vi "Pattern Rotation.vi"(1 "Rotation array":T1(array[cluster]), 2 "Rotation(degree)":dbl, 3 "Inkscape Image Size":cluster{"Width":dbl, "Height":dbl}) -> (0 "Rotated array":T1(array[cluster]))   [LabVIEW 2013]
uses:
  <vilib>/Analysis/coordinate.llb/2D Cartesian Coordinate Shift (Array).vi
  <vilib>/Analysis/coordinate.llb/2D Cartesian Coordinate Rotation (Array).vi
  <vilib>/Analysis/NI_AALPro.lvlib
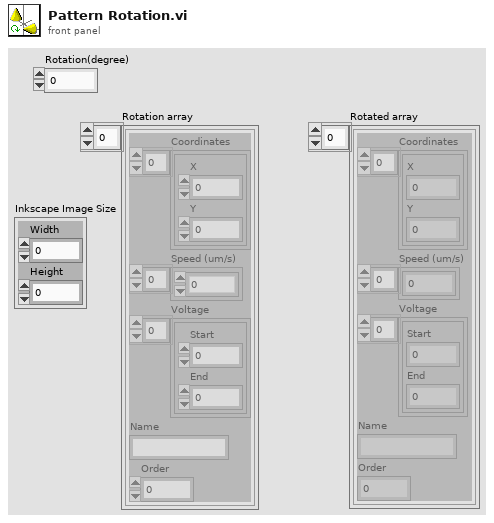
[diagram p1: front panel]
types:
  T1 = cluster{"Coordinates":cluster{"X":dbl, "Y":dbl}[], "Speed (um/s)":dbl[], "Voltage":cluster{"Start":dbl, "End":dbl}[], "Name":string, "Order":i32}[]
  T2 = cluster{"Coordinates":cluster{"X":dbl, "Y":dbl}[], "Speed (um/s)":dbl[], "Voltage":cluster{"Start":dbl, "End":dbl}[], "Name":string, "Order":i32}
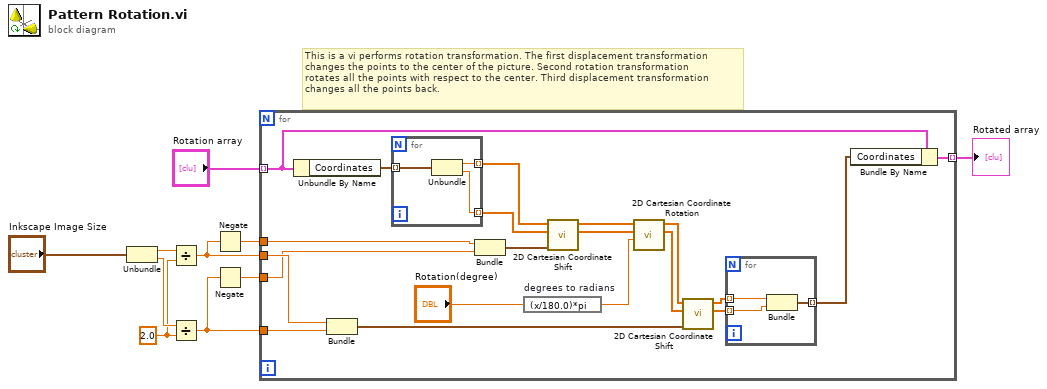
[diagram p0: block diagram]
diagram:
  w8 = 2.0 ("y")
  # "This is a vi performs rotation transformation. The first displacement transformation\nchanges the points to the center of the picture. Second rotation transformation \nrotates all the points with respect to the center. Third displacement transformation\nchanges all the points back."
  n1 = Unbundle("Inkscape Image Size") -> ("Width"=w10:dbl, "Height"=w9:dbl)
  n2 = Divide(x=w10, y=w8) -> (x/y=w6:dbl)
  n3 = Divide(x=w9, y=w8) -> (x/y=w4:dbl)
  n4 = Negate(x=w6) -> (-x=w7:dbl)
  n5 = Negate(x=w4) -> (-x=w5:dbl)
  n6 = for {
    tunnel: w7 -> [w30]
    tunnel: w6 -> [w29]
    tunnel: w5 -> [w28]
    tunnel: w4 -> [w27]
    tunnel: "Rotation array" -> [w13] mode=indexing
    tunnel: [w11] -> w1 mode=indexing
    n7 = Unbundle By Name(w13) -> ("Coordinates"=w16:cluster{"X":dbl, "Y":dbl}[])
    n8 = Bundle(w29, w27) -> (w19:cluster{dbl, dbl})  [unwired: 1 in]
    n9 = for {
      tunnel: w16 -> [w33] mode=indexing
      tunnel: [w32] -> w15 mode=indexing
      tunnel: [w31] -> w14 mode=indexing
      n10 = Unbundle(w33) -> ("X"=w32:dbl, "Y"=w31:dbl)
    }
    n11 = Bundle(w30, w28) -> (w20:cluster{dbl, dbl})  [unwired: 1 in]
    n12 = expression code="(x/180.0)*pi" "degrees to radians"("Rotation(degree)") -> (w17:dbl)
    n13 = call-poly <vilib>:"2D Cartesian Coordinate Shift.vi"("shift"=w20, "Y"=w14, "X"=w15) -> ("Y Out"=w21:dbl[], "X Out"=w22:dbl[])  [unwired: 6 in, 1 out]
    n14 = call-poly <vilib>:"2D Cartesian Coordinate Rotation.vi"("theta"=w17, "Y"=w21, "X"=w22) -> ("Y Out"=w25:dbl[], "X Out"=w26:dbl[])  [unwired: 6 in, 1 out]
    n15 = call-poly <vilib>:"2D Cartesian Coordinate Shift.vi"("shift"=w19, "Y"=w25, "X"=w26) -> ("Y Out"=w23:dbl[], "X Out"=w24:dbl[])  [unwired: 6 in, 1 out]
    n16 = for {
      tunnel: w24 -> [w36] mode=indexing
      tunnel: w23 -> [w35] mode=indexing
      tunnel: [w34] -> w12 mode=indexing
      n17 = Bundle("Numeric"=w36, "Numeric"=w35) -> (w34:cluster{"Numeric":dbl, "Numeric":dbl})  [unwired: 1 in]
    }
    n18 = Bundle By Name(cluster=w13, "Coordinates"=w12) -> (w11:T2)
  }
  "Rotated array" <- w1
